vi "GenerateCode.vi"(0 "机器码 2":string, 5 "注册码 2":string) -> (4 "鉴权通过":bool, 6 "参数配置":bool, 8 "参数生成":bool, 10 "强制操作":bool, 15 "数据保存":bool)   [LabVIEW 2013]
panel:
  out "长度":i32
  out "子字符串":string
  out "注册码 3":string
  out "Times":dbl
  out "Tip":string
  in  "退出":bool
  in  "注册":bool
  in  "注册码":string
  out "机器码":string
  out "字符串":string
  out "连接的字符串":string
  in  "簇":T1
  # "请输入注册码，请联系供应商获取!"
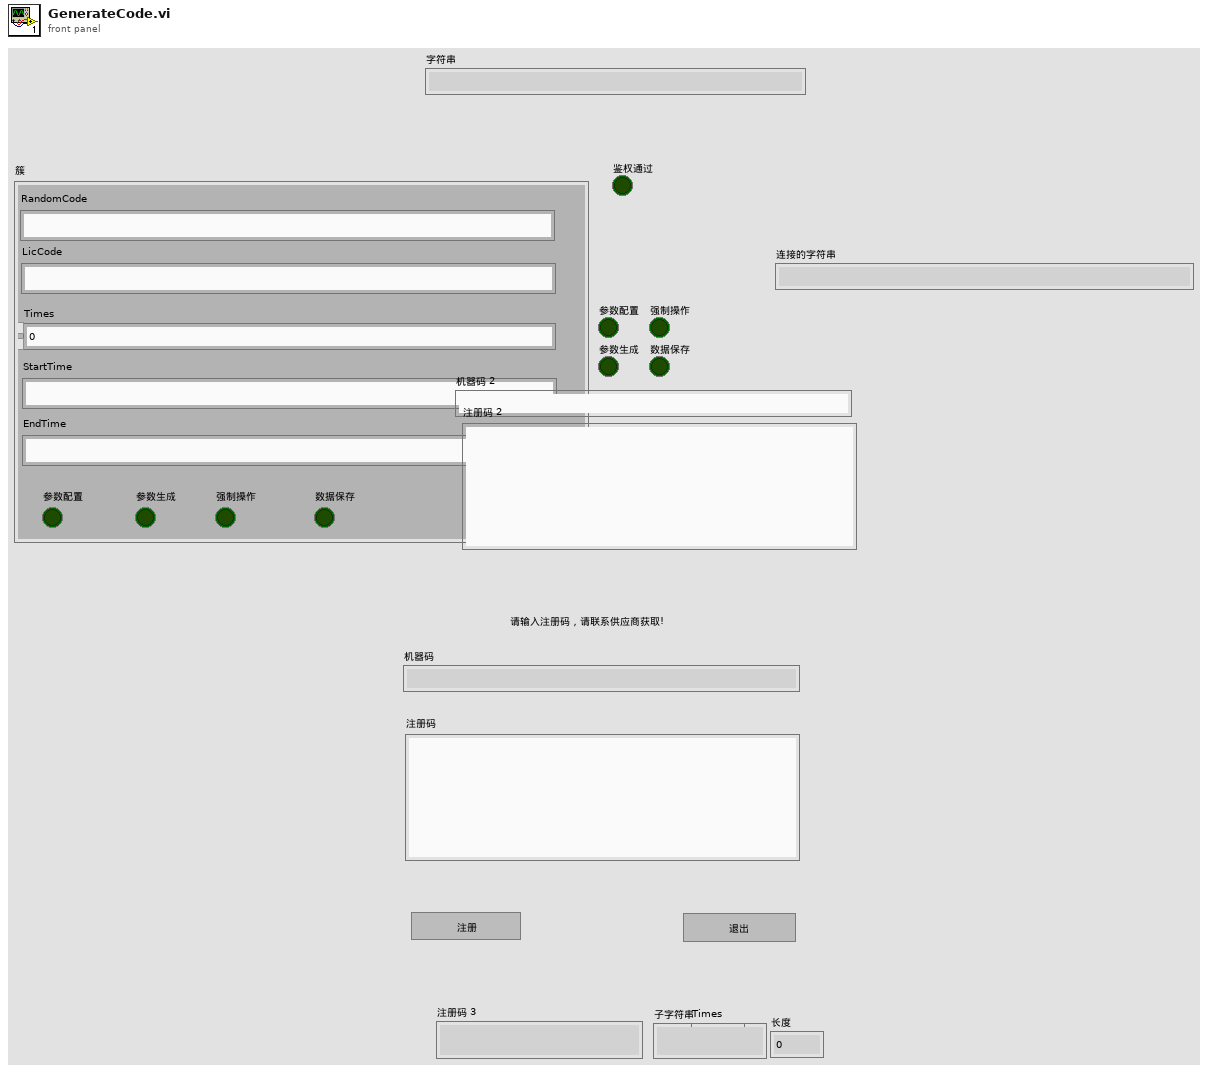
[diagram p1: front panel]
types:
  T1 = cluster{"RandomCode":string, "LicCode":string, "Times":dbl, "StartTime":string, "EndTime":string, "参数配置":bool, "参数生成":bool, "强制操作":bool, "数据保存":bool}
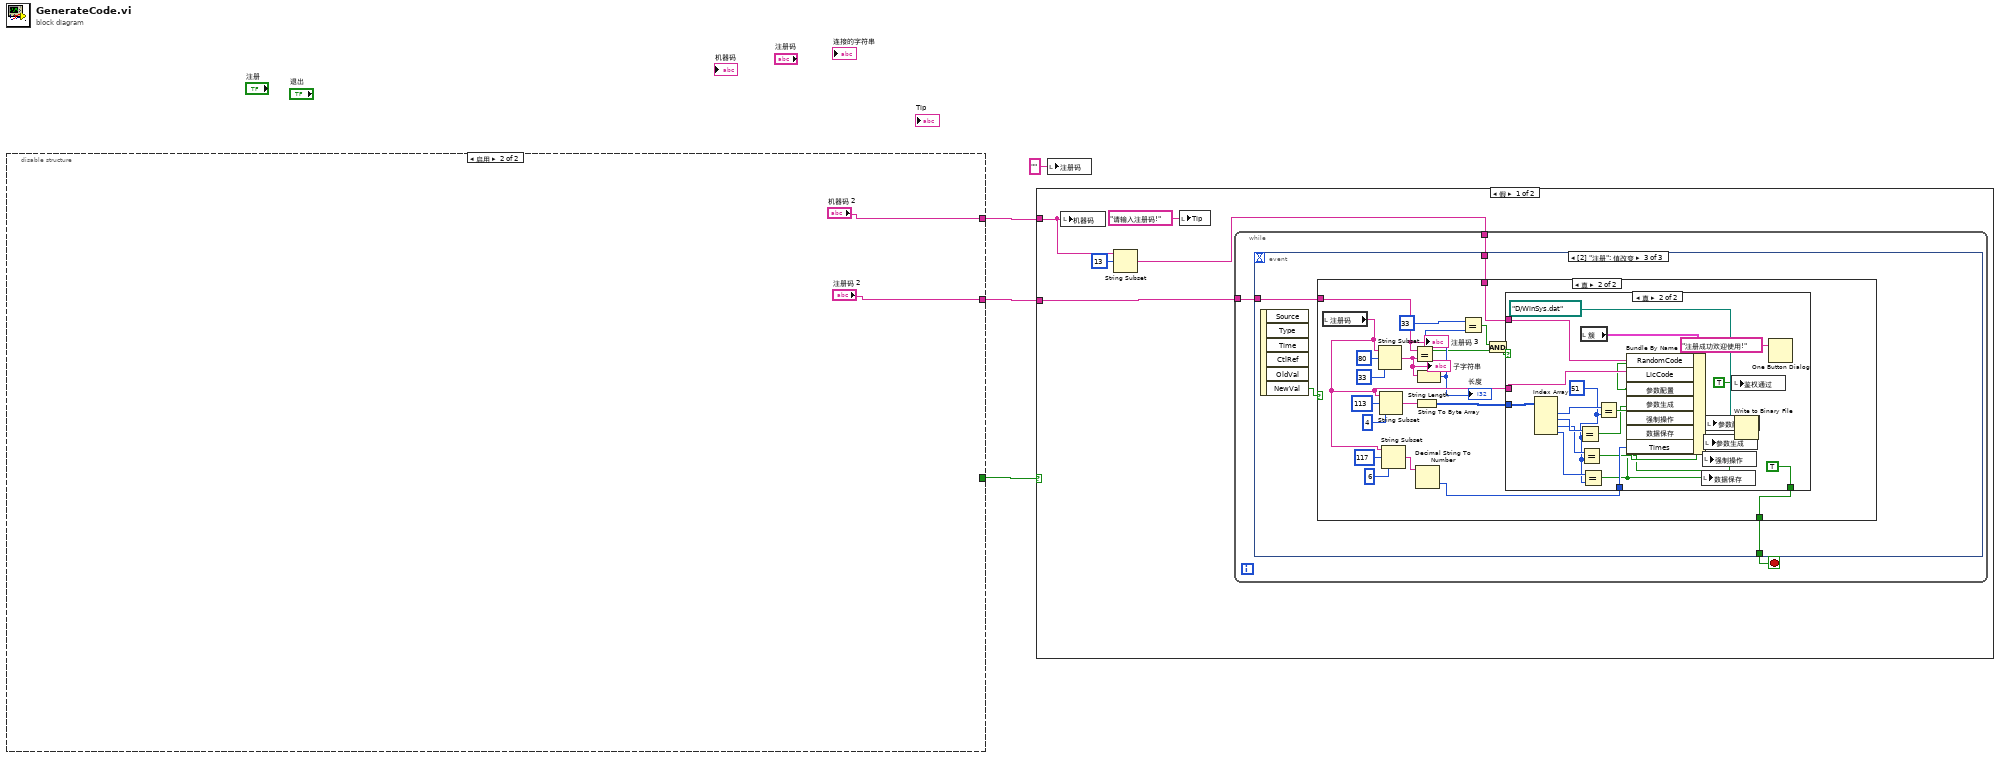
[diagram p0: block diagram]
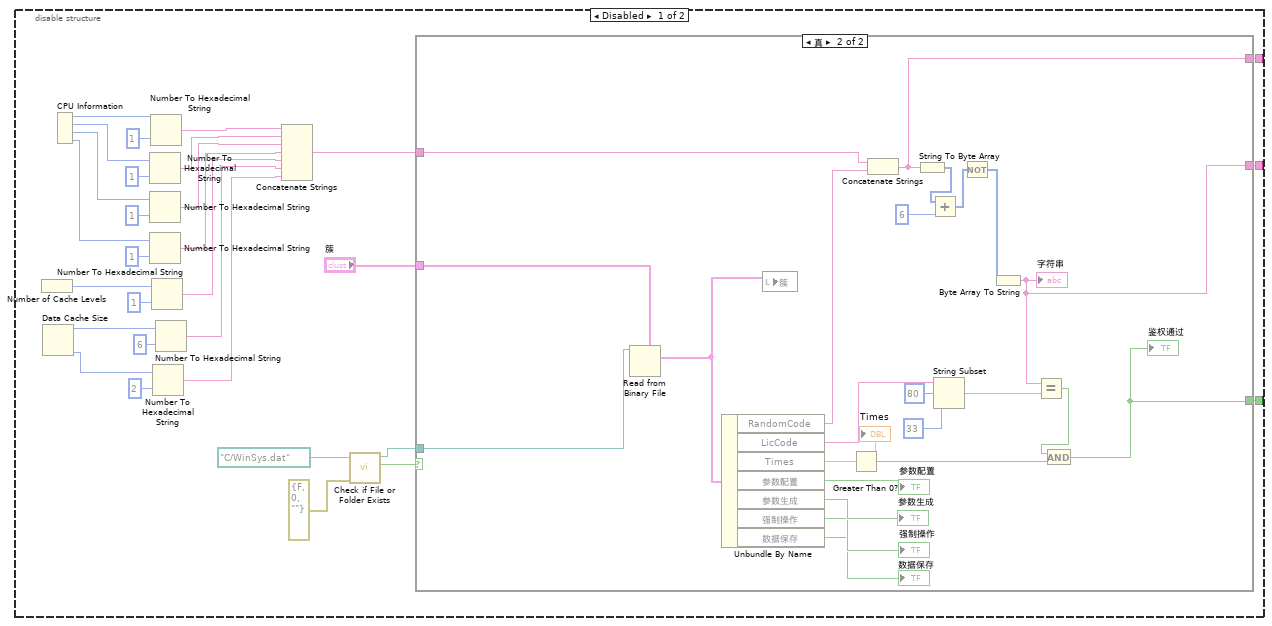
[diagram p2: hidden frame]
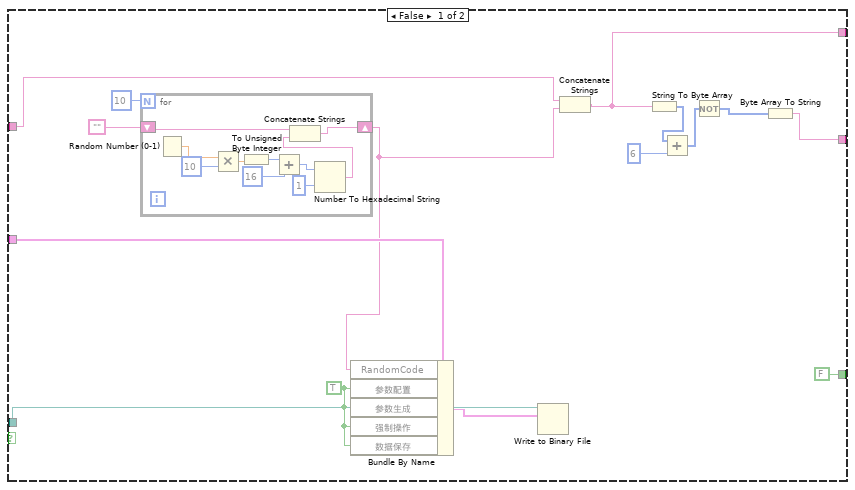
[diagram p3: hidden frame]
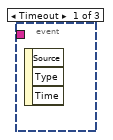
[diagram p4: hidden frame]
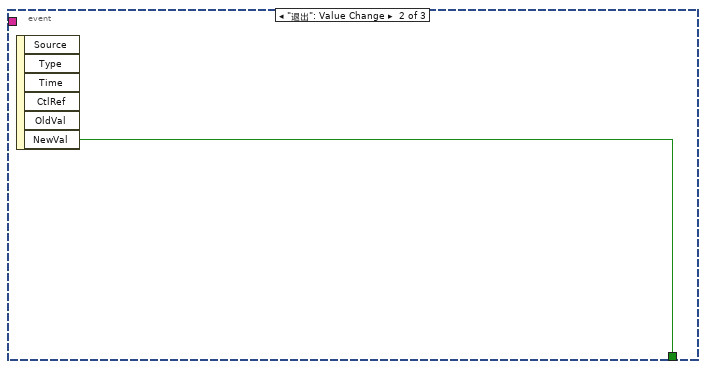
[diagram p5: hidden frame]
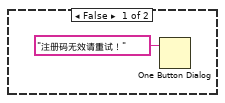
[diagram p7: hidden frame]
diagram:
  n1 = disable-structure shown="启用" {
    disable-tunnel: [w7 _] -> w4
    disable-tunnel: [w6 "注册码 2"] -> w3
    disable-tunnel: [w5 "机器码 2"] -> w2
    frame Disabled {
      n2 = Number of Cache Levels() -> (w19:i32)
      n3 = Data Cache Size() -> (4:w20:i32, 7:w22:i32)  [unwired: 1 in]
      n4 = CPU Information() -> (4:w10:i32, 5:w14:i32, 6:w15:i32, 7:w16:i32)
      n5 = Number To Hexadecimal String(1:i16 1 ("宽度(-)"), 2:w14) -> (0:w24:string)
      n6 = Number To Hexadecimal String(1:i16 1 ("宽度(-)"), 2:w15) -> (0:w25:string)
      n7 = Number To Hexadecimal String(1:i16 1 ("宽度(-)"), 2:w16) -> (0:w26:string)
      n8 = Number To Hexadecimal String(1:i16 1 ("宽度(-)"), 2:w10) -> (0:w23:string)
      n9 = Number To Hexadecimal String(1:i16 1 ("宽度(-)"), 2:w19) -> (0:w27:string)
      n10 = Number To Hexadecimal String(1:i16 2 ("宽度(-)"), 2:w22) -> (0:w29:string)
      n11 = Number To Hexadecimal String(1:i16 6 ("宽度(-)"), 2:w20) -> (0:w28:string)
      n12 = Concatenate Strings(w23, w24, w25, w26, w27, w28, w29) -> (w8:string)
      n13 = call <vilib>:"Check if File or Folder Exists.vi"("error in (no error)"=errorcluster {"status"=FALSE, "code"=0, "source"=""}, "path"=path "C:/WinSys.dat" ("文件（使用对话框）")) -> ("file or folder exists?"=w32:bool, "dup path"=w31:path)  [unwired: 7 in, 1 out]
      n14 = case shown="真" w32 {
        tunnel: w31 -> [w48 w80]
        tunnel: "簇" -> [w44 w79]
        tunnel: w8 -> [w41 w73]
        tunnel: [FALSE w65] -> w7
        tunnel: [w36 w64] -> w6
        tunnel: [w35 w59] -> w5
        frame False {
          w43 = TRUE ("参数配置")
          n15 = for {
            N: 10 -> [_]
            shift-right: [w50] -> w40
            shift-left: "" -> [w51]
            n16 = Random Number (0-1)() -> (number: 0 to 1=w58:dbl)
            n17 = Multiply(x=w58, y=u8 10) -> (x*y=w56:dbl)
            n18 = To Unsigned Byte Integer(number=w56) -> (unsigned 8bit integer=w54:u8)
            n19 = Add(x=w54, y=u8 16) -> (x+y=w52:u8)
            n20 = Number To Hexadecimal String(1:i16 1 ("宽度(-)"), 2:w52) -> (0:w49:string)
            n21 = Concatenate Strings(w51, w49) -> (w50:string)
          }
          n22 = Bundle By Name(cluster=w44, "RandomCode"=w40, "参数配置"=w43, "参数生成"=w43, "强制操作"=w43, "数据保存"=w43) -> (w47:T1)
          n23 = Write to Binary File(file (use dialog)=w48, data=w47) -> ()  [unwired: 4 in, 3 out]
          n24 = Concatenate Strings(w41, w40) -> (w35:string)
          n25 = String To Byte Array(string=w35) -> (unsigned byte array=w39:u8[])
          n26 = Add(x=w39, y=u8 6) -> (x+y=w37:u8[])
          n27 = Not(x=w37) -> ()  [unwired: 1 out]
          n28 = Byte Array To String(unsigned byte array=w37) -> (string=w36:string)
        }
        frame True {
          n29 = Read from Binary File(5:w79, 11:w80) -> (2:w78:T1)  [unwired: 4 in, 3 out]
          n30 = Unbundle By Name(w78) -> ("RandomCode"=w74:string, "LicCode"=w77:string, "Times"=w68:dbl, "参数配置"=→"参数配置":bool, "参数生成"=→"参数生成":bool, "强制操作"=→"强制操作":bool, "数据保存"=→"数据保存":bool)
          "Times" <- w68
          n31 = local write "簇"(w78) -> ()
          n32 = Greater Than 0?(x=w68) -> (x > 0?=w66:bool)
          n33 = Concatenate Strings(w73, w74) -> (w59:string)
          n34 = String To Byte Array(string=w59) -> (unsigned byte array=w72:u8[])
          n35 = Add(x=w72, y=u8 6) -> (x+y=w70:u8[])
          n36 = String Subset(string=w77, offset (0)=80 ("偏移量(0)"), length (rest)=33 ("长度（剩余）")) -> (substring=w69:string)
          n37 = Not(x=w70) -> ()  [unwired: 1 out]
          n38 = Byte Array To String(unsigned byte array=w70) -> (string=w64:string)
          "字符串" <- w64
          n39 = Equal?(x=w64, y=w69) -> (x = y?=w67:bool)
          n40 = And(x=w67, y=w66) -> (x .and. y?=w65:bool)
          "鉴权通过" <- w65
        }
      }
    }
    frame Enabled {
    }
  }
  n41 = case shown="假" w4 {
    tunnel: w3 -> [w87 _]
    tunnel: w2 -> [w85 _]
    frame False {
      n42 = local write "机器码"(w85) -> ()
      n43 = String Subset(string=w85, offset (0)=13 ("偏移量(0)")) -> (substring=w83:string)  [unwired: 1 in]
      n44 = local write "Tip"("请输入注册码!" ("Tip")) -> ()
      n45 = while {
        tunnel: w87 -> [w90]
        tunnel: w83 -> [w88]
        stop <- w89 stop-if-true
        n46 = event shown="[2] \"注册\": 值改变" {
          selector: _ -> [_ _ _]
          dyn-events: _ -> [_ _ _]
          timeout: _ -> [_ _ _]
          tunnel: w90 -> [_ _ w95]
          tunnel: [_ w91 w94] -> w89
          tunnel: w88 -> [_ _ w93]
          event Timeout {
            n47 = event-data() -> ()  [unwired: 1 in, 3 out]
          }
          event "退出": Value Change {
            n48 = event-data() -> ("NewVal"=w91:bool)  [unwired: 1 in, 5 out]
          }
          event "注册": Value Change {
            n49 = event-data() -> ("NewVal"=w92:bool)  [unwired: 1 in, 5 out]
            n50 = case shown="真" w92 {
              tunnel: w95 -> [_ w113]
              tunnel: [_ w103] -> w94
              tunnel: w93 -> [_ w96]
              frame False {
              }
              frame True {
                n51 = local read "注册码"() -> (w106:string)
                n52 = String Subset(string=w106, offset (0)=80 ("偏移量(0)"), length (rest)=33 ("长度（剩余）")) -> (substring=w102:string)
                "子字符串" <- w102
                n53 = String Subset(string=w106, offset (0)=113 ("偏移量(0)"), length (rest)=4 ("长度（剩余）")) -> (substring=w110:string)
                n54 = String Subset(string=w106, offset (0)=117 ("偏移量(0)"), length (rest)=6 ("长度（剩余）")) -> (substring=w105:string)
                n55 = Equal?(x=w113, y=w102) -> (x = y?=w98:bool)
                n56 = String To Byte Array(string=w110) -> (unsigned byte array=w109:u8[])
                n57 = Decimal String To Number(string=w105) -> (number=w104:i32)  [unwired: 2 in, 1 out]
                n58 = String Length(string=w102) -> (length=w101:i32)
                "长度" <- w101
                n59 = Equal?(x=33, y=w101) -> (x = y?=w99:bool)
                n60 = And(x=w99, y=w98) -> (x .and. y?=w97:bool)
                n61 = case shown="真" w97 {
                  tunnel: w109 -> [_ w132]
                  tunnel: w106 -> [_ w126]
                  tunnel: w104 -> [_ w125]
                  tunnel: [_ TRUE ("新值")] -> w103
                  tunnel: w96 -> [_ w117]
                  frame False {
                    n62 = One Button Dialog(message="注册码无效请重试！" ("消息")) -> ()  [unwired: 1 in, 1 out]
                  }
                  frame True {
                    w127 = 51 ("索引")
                    n63 = Index Array(array=w132) -> (element #1=w131:u8, element #2=w130:u8, element #3=w129:u8, element #4=w128:u8)  [unwired: 4 in]
                    n64 = Equal?(x=w130, y=w127) -> (x = y?=w120:bool)
                    n65 = Equal?(x=w129, y=w127) -> (x = y?=w119:bool)
                    n66 = local read "簇"() -> (w133:T1)
                    n67 = Equal?(x=w128, y=w127) -> (x = y?=w118:bool)
                    n68 = Equal?(x=w131, y=w127) -> (x = y?=w121:bool)
                    n69 = Bundle By Name(cluster=w133, "RandomCode"=w117, "LicCode"=w126, "参数配置"=w121, "参数生成"=w120, "强制操作"=w119, "数据保存"=w118, "Times"=w125) -> (w135:T1)
                    n70 = local write "数据保存"(w118) -> ()
                    n71 = local write "强制操作"(w119) -> ()
                    n72 = local write "参数生成"(w120) -> ()
                    n73 = local write "参数配置"(w121) -> ()
                    n74 = local write "鉴权通过"(TRUE ("鉴权通过")) -> ()
                    n75 = Write to Binary File(file (use dialog)=path "D:/WinSys.dat" ("文件（使用对话框）"), data=w135) -> ()  [unwired: 4 in, 3 out]
                    n76 = One Button Dialog(message="注册成功欢迎使用!" ("消息")) -> ()  [unwired: 1 in, 1 out]
                  }
                }
                "注册码 3" <- w113
              }
            }
          }
        }
      }
    }
    frame True {
    }
  }
  n77 = local write "注册码"("" ("注册码")) -> ()
